vi "Close Connection.vi"(8 "error in (no error)":errorcluster, 11 "NXP in":refnum<class "NXP.lvclass">) -> (0 "error out":errorcluster, 3 "NXP out":refnum<class "NXP.lvclass">)   [LabVIEW 2020, in "NXP.lvclass"]
uses:
  NXP.lvclass
  NXP.lvclass/NXP.ctl
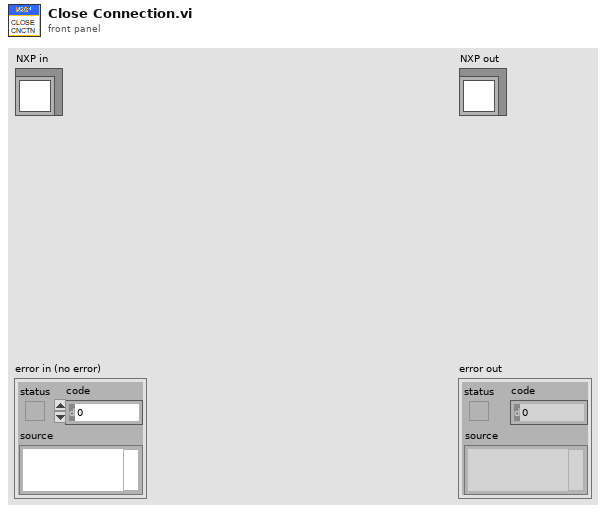
[diagram p1: front panel]
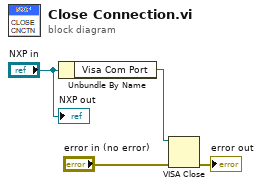
[diagram p0: block diagram]
diagram:
  n1 = Unbundle By Name("NXP in") -> ("Visa Com Port"=w4:refnum<visa-resource-name>)
  n2 = VISA Close(VISA resource name=w4, error in (no error)="error in (no error)") -> (error out=→"error out":errorcluster)
  "NXP out" <- "NXP in"
